vi "TIRFLockGetVotage.vi"(7 "error in (no error)":errorcluster, 10 "Config In":T1={"Hardware Configuration"={"Camera Configuration"={"Setting"={"Expouse"=0.0, "Frames"=0.0, "Interval"=0.0, "ROI"={"x"=0.0, "y"=0.0, "width"=0.0, "height"=0.0}, "Binning"={"Binning X"=0.0, "Binning Y"=0.0}}, "Resource"={"CameraRef"=refnum, "LibraryRef"=refnum, "ImagesArray"=[]}}, "Stages Configuration"={"Resource"={"NanoStage Ref"=0, "MicroStage Ref"=0, "TirfLock Ref"=0}, "SettingValues"={"NanoState"={"Time"=0.0, "X"=0.0, "Y"=0.0, "Z"=0.0}, "MicroState"={"Time 2"=0.0, "Z"=0.0, "IsEPISet?"=FALSE}, "TirfLock"={"Time"=0.0, "X"=0.0, "Y"=0.0, "Sum"=0.0, "Calbrate"=0.0, "LockedTarget"=0.0, "Kp"=0.0, "Ki"=0.0, "Avg"=0.0}}}, "Lasers Configuration"={"SettingValues"={"405 Power"=0.0, "488 Power"=0.0, "532 Power"=0.0, "561 Power"=0.0, "647 Power"=0.0, "785 Power"=0.0}, "Resource"={"Library Ref"=refnum, "Lasers Ref"={"405 Ref"=refnum, "488 Ref"=refnum, "532 Ref"=refnum, "561 Ref"=refnum, "647 Ref"=refnum, "785 Ref"=refnum}}}}, "Logging Configuration"={"Log File Base Folder"=path "", "FileSurfix"="", "TiffFileFullPath"=path "", "TimeStampFile Ref"=refnum, "NoteFileRef"=refnum, "QuickNoteInfo"=""}, "HardWare Status"={"CameraAndStages"={"Camera"=FALSE, "NanoStage"=FALSE, "MicroStage"=FALSE, "TIRFLock"=FALSE}, "Lasers"={"IsConnected"={"405"=FALSE, "488"=FALSE, "532"=FALSE, "561"=FALSE, "647"=FALSE, "785"=FALSE}, "IsOpened"={"405"=FALSE, "488"=FALSE, "532"=FALSE, "561"=FALSE, "647"=FALSE, "785"=FALSE}}}, "CallBack Ref"={"LiveAcq callback Ref"=refnum, "AlbumAcq callback Ref"=refnum, "SequenceAcq callback Ref"=refnum, "Camera Status callback Ref"=refnum}, "Acqusition Control"={"Images Saving"={"StreamToDisk?"=FALSE, "SingleStack?"=FALSE, "Alert when finish?"=FALSE}, "Debug"={"Global Debug"=FALSE, "Global Debug Value"=0.0}}, "Runtime Parameters"={"Scale Bar"=TRUE, "ScaleBarSize"=10.0, "XYIncreatement+"=40.0, "ZIncreatement++"=5.0, "Autostretch"=FALSE, "Binning"=0.0, "ZIncreatement+"=0.2, "MicroStage+"=100.0, "Exposure"=200.0, "Interval"=200.0, "XYIncreatement++"=80.0, "CaptureFrame"=500.0}} {"Runtime Parameters"."CaptureFrame" format="%#_13g"; "Runtime Parameters"."XYIncreatement++" format="%#_13g"; "Runtime Parameters"."Interval" format="%#_13g"; "Runtime Parameters"."Exposure" format="%#_13g"; "Runtime Parameters"."MicroStage+" format="%#_13g"; "Runtime Parameters"."ZIncreatement+" format="%#_13g"; "Runtime Parameters"."Binning" format="%#_13g"; "Runtime Parameters"."ZIncreatement++" format="%#_13g"; "Runtime Parameters"."XYIncreatement+" format="%#_13g"; "Runtime Parameters"."ScaleBarSize" format="%#_13g"; "Hardware Configuration"."Lasers Configuration"."SettingValues"."785 Power" format="%.1f"; "Hardware Configuration"."Lasers Configuration"."SettingValues"."647 Power" format="%.1f"; "Hardware Configuration"."Lasers Configuration"."SettingValues"."561 Power" format="%.1f"}) -> (0 "error out":errorcluster, 2 "TirfLock":cluster{"Time":dbl, "X":dbl, "Y":dbl, "Sum":dbl}, 3 "Config dup":T1={"Hardware Configuration"={"Camera Configuration"={"Setting"={"Expouse"=0.0, "Frames"=0.0, "Interval"=0.0, "ROI"={"x"=0.0, "y"=0.0, "width"=0.0, "height"=0.0}, "Binning"={"Binning X"=0.0, "Binning Y"=0.0}}, "Resource"={"CameraRef"=refnum, "LibraryRef"=refnum, "ImagesArray"=[]}}, "Stages Configuration"={"Resource"={"NanoStage Ref"=0, "MicroStage Ref"=0, "TirfLock Ref"=0}, "SettingValues"={"NanoState"={"Time"=0.0, "X"=0.0, "Y"=0.0, "Z"=0.0}, "MicroState"={"Time 2"=0.0, "Z"=0.0, "IsEPISet?"=FALSE}, "TirfLock"={"Time"=0.0, "X"=0.0, "Y"=0.0, "Sum"=0.0, "Calbrate"=0.0, "LockedTarget"=0.0, "Kp"=0.0, "Ki"=0.0, "Avg"=0.0}}}, "Lasers Configuration"={"SettingValues"={"405 Power"=0.0, "488 Power"=0.0, "532 Power"=0.0, "561 Power"=0.0, "647 Power"=0.0, "785 Power"=0.0}, "Resource"={"Library Ref"=refnum, "Lasers Ref"={"405 Ref"=refnum, "488 Ref"=refnum, "532 Ref"=refnum, "561 Ref"=refnum, "647 Ref"=refnum, "785 Ref"=refnum}}}}, "Logging Configuration"={"Log File Base Folder"=path "", "FileSurfix"="", "TiffFileFullPath"=path "", "TimeStampFile Ref"=refnum, "NoteFileRef"=refnum, "QuickNoteInfo"=""}, "HardWare Status"={"CameraAndStages"={"Camera"=FALSE, "NanoStage"=FALSE, "MicroStage"=FALSE, "TIRFLock"=FALSE}, "Lasers"={"IsConnected"={"405"=FALSE, "488"=FALSE, "532"=FALSE, "561"=FALSE, "647"=FALSE, "785"=FALSE}, "IsOpened"={"405"=FALSE, "488"=FALSE, "532"=FALSE, "561"=FALSE, "647"=FALSE, "785"=FALSE}}}, "CallBack Ref"={"LiveAcq callback Ref"=refnum, "AlbumAcq callback Ref"=refnum, "SequenceAcq callback Ref"=refnum, "Camera Status callback Ref"=refnum}, "Acqusition Control"={"Images Saving"={"StreamToDisk?"=FALSE, "SingleStack?"=FALSE, "Alert when finish?"=FALSE}, "Debug"={"Global Debug"=FALSE, "Global Debug Value"=0.0}}, "Runtime Parameters"={"Scale Bar"=TRUE, "ScaleBarSize"=10.0, "XYIncreatement+"=40.0, "ZIncreatement++"=5.0, "Autostretch"=FALSE, "Binning"=0.0, "ZIncreatement+"=0.2, "MicroStage+"=100.0, "Exposure"=200.0, "Interval"=200.0, "XYIncreatement++"=80.0, "CaptureFrame"=500.0}} {"Runtime Parameters"."CaptureFrame" format="%#_13g"; "Runtime Parameters"."XYIncreatement++" format="%#_13g"; "Runtime Parameters"."Interval" format="%#_13g"; "Runtime Parameters"."Exposure" format="%#_13g"; "Runtime Parameters"."MicroStage+" format="%#_13g"; "Runtime Parameters"."ZIncreatement+" format="%#_13g"; "Runtime Parameters"."Binning" format="%#_13g"; "Runtime Parameters"."ZIncreatement++" format="%#_13g"; "Runtime Parameters"."XYIncreatement+" format="%#_13g"; "Runtime Parameters"."ScaleBarSize" format="%#_13g"; "Hardware Configuration"."Lasers Configuration"."SettingValues"."785 Power" format="%.1f"; "Hardware Configuration"."Lasers Configuration"."SettingValues"."647 Power" format="%.1f"; "Hardware Configuration"."Lasers Configuration"."SettingValues"."561 Power" format="%.1f"})   [LabVIEW 2020]
doc: "Generates sample waveforms according to the signal type in the HW Config input."
uses:
  Settings/System Running Settings.ctl
  Support/Hardware Configuration.ctl
  Support/Camera Configuration.ctl
  controls/ROI.ctl
  D:/Daguan/Development/RM21-MMicrosopeSource/HardwareAdapter/Camera/Dependencies/PVCamNET.dll
  Camera/Dependencies/PVCamNET.dll
  <vilib>/vision/Image Controls.llb/IMAQ Image.ctl
  D:/Daguan/Development/RM21-MMicrosopeSource/HardwareAdapter/Lasers/Dependencies/Oxxius_Boxx.dll
  Lasers/Dependencies/Oxxius_Boxx.dll
  Logging/Logging Configuration.ctl
  controls/DeviceStatusCtl.ctl
  controls/CallBack Refs.ctl
  Acquisition/Acquisition Control.ctl
  controls/Runtime Parameters.ctl
  Global.vi
  Logging/Logging.lvlib
  Settings/Settings.lvlib
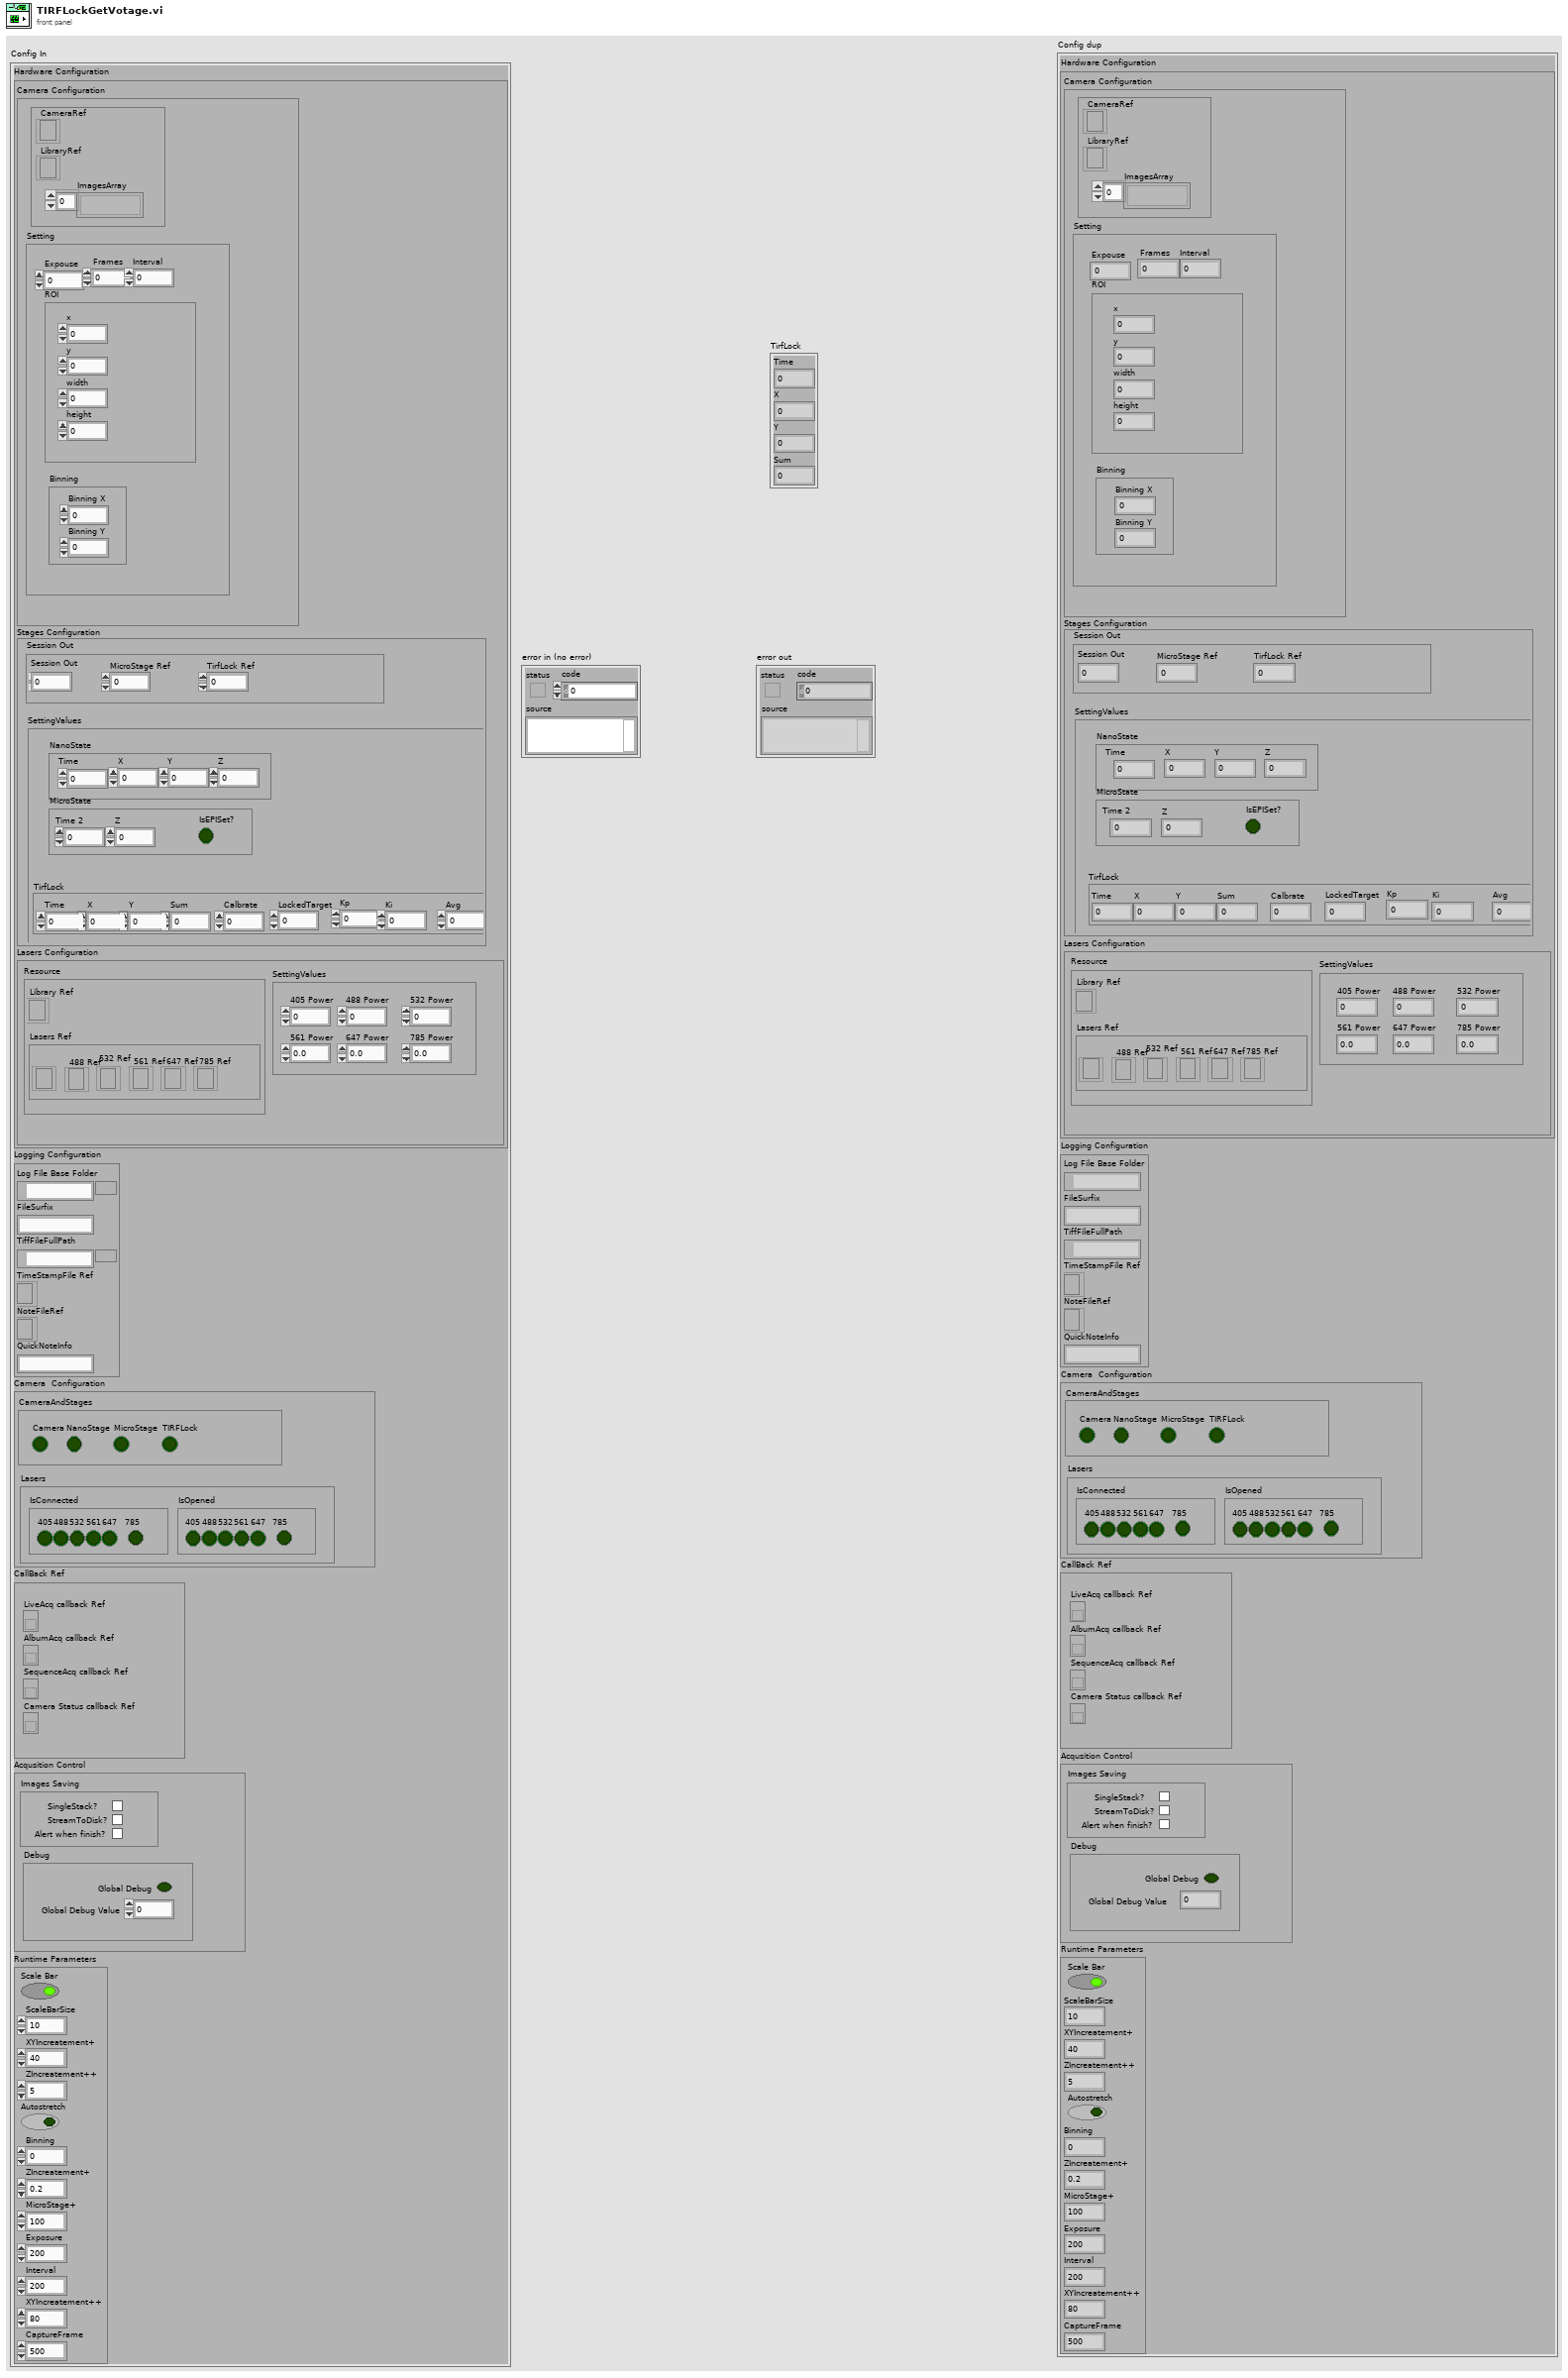
[diagram p1: front panel]
types:
  T1 = typedef "Settings.lvlib/System Running Settings.ctl" = cluster{"Hardware Configuration":T2, "Logging Configuration":T6, "HardWare Status":cluster{"CameraAndStages":T7, "Lasers":cluster{"IsConnected":cluster{"405":bool, "488":bool, "532":bool, "561":bool, "647":bool, "785":bool}, "IsOpened":cluster{"405":bool, "488":bool, "532":bool, "561":bool, "647":bool, "785":bool}}}, "CallBack Ref":T8, "Acqusition Control":T9, "Runtime Parameters":T10}
  T2 = typedef "Hardware Configuration.ctl" = cluster{"Camera Configuration":T3, "Stages Configuration":cluster{"Resource":cluster{"NanoStage Ref":i32, "MicroStage Ref":i32, "TirfLock Ref":i32}, "SettingValues":cluster{"NanoState":cluster{"Time":dbl, "X":dbl, "Y":dbl, "Z":dbl}, "MicroState":cluster{"Time 2":dbl, "Z":dbl, "IsEPISet?":bool}, "TirfLock":cluster{"Time":dbl, "X":dbl, "Y":dbl, "Sum":dbl, "Calbrate":dbl, "LockedTarget":dbl, "Kp":dbl, "Ki":dbl, "Avg":dbl}}}, "Lasers Configuration":cluster{"SettingValues":cluster{"405 Power":sgl, "488 Power":sgl, "532 Power":sgl, "561 Power":sgl, "647 Power":sgl, "785 Power":sgl}, "Resource":cluster{"Library Ref":refnum<k24>, "Lasers Ref":cluster{"405 Ref":refnum<k24>, "488 Ref":refnum<k24>, "532 Ref":refnum<k24>, "561 Ref":refnum<k24>, "647 Ref":refnum<k24>, "785 Ref":refnum<k24>}}}}
  T3 = typedef "Camera Configuration.ctl" = cluster{"Setting":cluster{"Expouse":dbl, "Frames":dbl, "Interval":dbl, "ROI":T4, "Binning":cluster{"Binning X":dbl, "Binning Y":dbl}}, "Resource":cluster{"CameraRef":refnum<k24>, "LibraryRef":refnum<k24>, "ImagesArray":T5[]}}
  T4 = typedef "ROI.ctl" = cluster{"x":dbl, "y":dbl, "width":dbl, "height":dbl}
  T5 = typedef "IMAQ Image.ctl" = refnum<image>
  T6 = typedef "Logging.lvlib/Logging Configuration.ctl" = cluster{"Log File Base Folder":path, "FileSurfix":string, "TiffFileFullPath":path, "TimeStampFile Ref":refnum<file>, "NoteFileRef":refnum<file>, "QuickNoteInfo":string}
  T7 = typedef "DeviceStatusCtl.ctl" = cluster{"Camera":bool, "NanoStage":bool, "MicroStage":bool, "TIRFLock":bool}
  T8 = typedef "CallBack Refs.ctl" = cluster{"LiveAcq callback Ref":refnum<k27>, "AlbumAcq callback Ref":refnum<k27>, "SequenceAcq callback Ref":refnum<k27>, "Camera Status callback Ref":refnum<k27>}
  T9 = typedef "Acquisition Control.ctl" = cluster{"Images Saving":cluster{"StreamToDisk?":bool, "SingleStack?":bool, "Alert when finish?":bool}, "Debug":cluster{"Global Debug":bool, "Global Debug Value":dbl}}
  T10 = typedef "Runtime Parameters.ctl" = cluster{"Scale Bar":bool, "ScaleBarSize":dbl, "XYIncreatement+":dbl, "ZIncreatement++":dbl, "Autostretch":bool, "Binning":dbl, "ZIncreatement+":dbl, "MicroStage+":dbl, "Exposure":dbl, "Interval":dbl, "XYIncreatement++":dbl, "CaptureFrame":dbl}
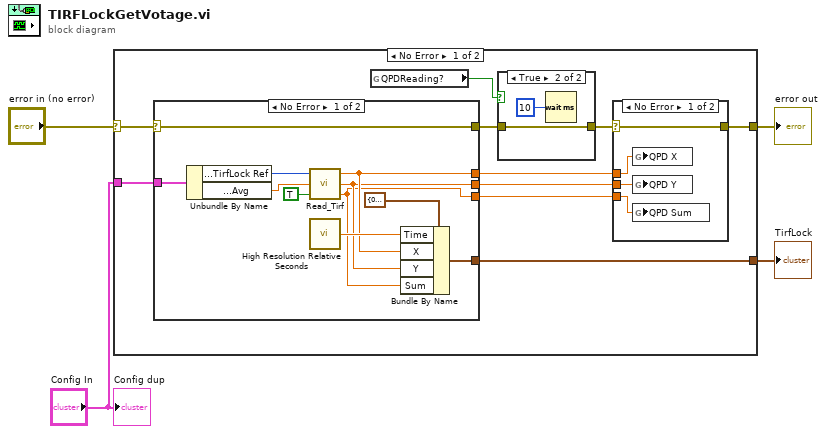
[diagram p0: block diagram]
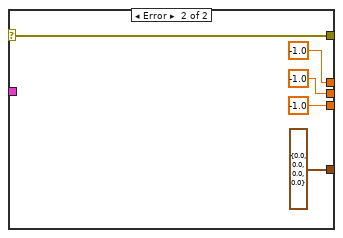
[diagram p2: hidden frame]
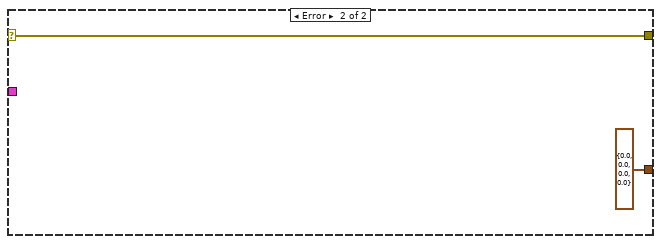
[diagram p5: hidden frame]
diagram:
  n1 = case shown="No Error" "error in (no error)" {
    selector: "error in (no error)" -> [w7 w39]
    tunnel: "Config In" -> [w13 _]
    tunnel: [w14 cluster{"Time":dbl, "X":dbl, "Y":dbl, "Sum":dbl} {"Time"=0.0, "X"=0.0, "Y"=0.0, "Sum"=0.0} ("RawImage")] -> w3
    tunnel: [w8 w39] -> w1
    frame No Error {
      n2 = case shown="No Error" w7 {
        selector: w7 -> [w15 w26]
        tunnel: [w25 cluster{"Time":dbl, "X":dbl, "Y":dbl, "Sum":dbl} {"Time"=0.0, "X"=0.0, "Y"=0.0, "Sum"=0.0} ("RawImage")] -> w14
        tunnel: w13 -> [w24 _]
        tunnel: [w18 -1.0 ("coerced(x)")] -> w12
        tunnel: [w17 -1.0 ("coerced(y)")] -> w11
        tunnel: [w16 -1.0 ("coerced(sum)")] -> w10
        tunnel: [w15 w26] -> w6
        frame No Error {
          n3 = Unbundle By Name(w24) -> ("Hardware Configuration.Stages Configuration.Resource.TirfLock Ref"=w23:i32, "Hardware Configuration.Stages Configuration.SettingValues.TirfLock.Avg"=w22:dbl)
          n4 = call "Read_Tirf.vi"("Display"=TRUE, "Averages"=w22, "Tirf-Handle"=w23) -> ("coerced(sum)"=w16:dbl, "coerced(y)"=w17:dbl, "coerced(x)"=w18:dbl)
          n5 = call <vilib>:"High Resolution Relative Seconds.vi"() -> ("relative seconds"=w19:dbl)
          n6 = Bundle By Name(cluster=cluster{"Time":dbl, "X":dbl, "Y":dbl, "Sum":dbl} {"Time"=0.0, "X"=0.0, "Y"=0.0, "Sum"=0.0} ("RawImage"), "Time"=w19, "X"=w18, "Y"=w17, "Sum"=w16) -> (w25:cluster{"Time":dbl, "X":dbl, "Y":dbl, "Sum":dbl})
        }
        frame Error {
        }
      }
      n7 = global read "Global.vi" "QPDReading?"() -> (w5:bool)
      n8 = case shown="True" w5 {
        tunnel: w6 -> [w31 w32]
        tunnel: [w31 w32] -> w9
        frame False {
        }
        frame True {
          n9 = Wait (ms)(milliseconds to wait=u32 10) -> ()  [unwired: 1 out]
        }
      }
      n10 = case shown="No Error" w9 {
        selector: w9 -> [w34 w38]
        tunnel: w10 -> [w37 _]
        tunnel: w11 -> [w36 _]
        tunnel: w12 -> [w35 _]
        tunnel: [w34 w38] -> w8
        frame No Error {
          n11 = global write "Global.vi" "QPD X"(w35) -> ()
          n12 = global write "Global.vi" "QPD Y"(w36) -> ()
          n13 = global write "Global.vi" "QPD Sum"(w37) -> ()
        }
        frame Error {
        }
      }
    }
    frame Error {
    }
  }
  "error out" <- w1
  "TirfLock" <- w3
  "Config dup" <- "Config In"
